vi "TCP Named Service - Server.vi"() -> ()   [LabVIEW 2013]
doc: "创建一个命名服务并在第一个可用端口侦听。当客户端连接该服务时，将发送一个响应字符串至客户端。"
panel:
  in  "发送的消息":string="当前正从客户端%s（端口%d）访问TCP Named Service - Server.vi。"
  in  "停止":bool
  # "概述：演示使用TCP函数初始化可向客户端VI发送数据的命名TCP服务。\n操作步骤：\n1. 运行VI。\n2. 打开TCP Named Service - Client.vi并按前面板上的说明操作。\n3. 单击停止可停止VI。"
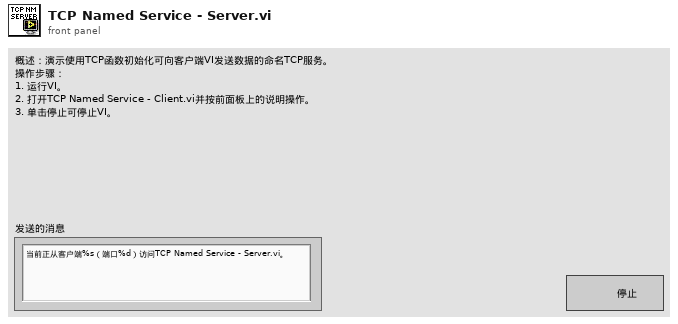
[diagram p1: front panel]
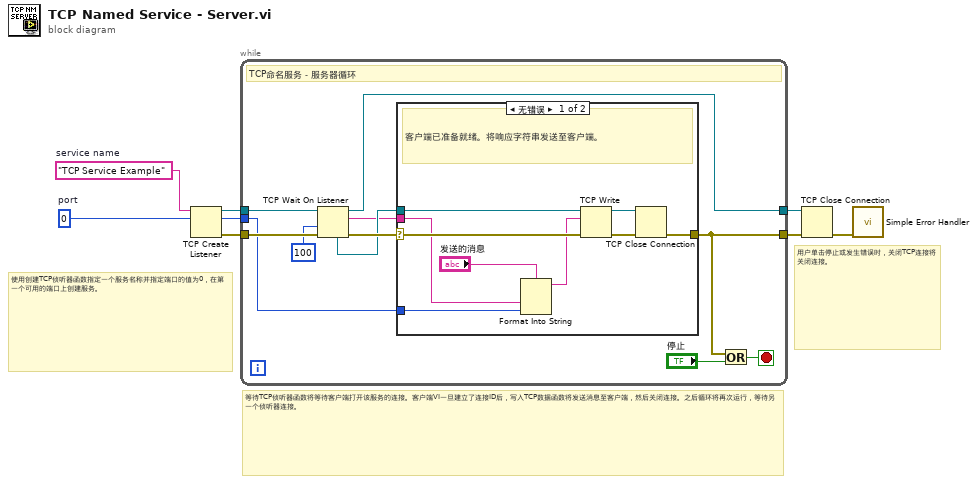
[diagram p0: block diagram]
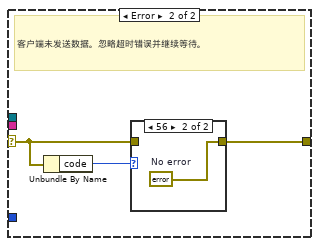
[diagram p2: hidden frame]
diagram:
  w2 = u16 0  # port
  w1 = "TCP Service Example"  # service name
  # "用户单击停止或发生错误时，关闭TCP连接将关闭连接。"
  # "等待TCP侦听器函数将等待客户端打开该服务的连接。客户端VI一旦建立了连接ID后，写入TCP数据函数将发送消息至客户端，然后关闭连接。之后循环将再次运行，等待另一个侦听器连接。"
  # "使用创建TCP侦听器函数指定一个服务名称并指定端口的值为0，在第一个可用的端口上创建服务。"
  n1 = TCP Create Listener(10:w2, 11:w1) -> (0:w7:errorcluster, 2:w4:u16, 3:w8:refnum<k5>)  [unwired: 3 in]
  n2 = while {
    tunnel: [w12] -> w5
    tunnel: w8 -> [w19]
    tunnel: w7 -> [w17]
    tunnel: [w9] -> w6
    tunnel: w4 -> [w15]
    stop <- w14 stop-if-true
    # "TCP命名服务－服务器循环"
    n3 = TCP Wait On Listener(8:w17, 9:100 ("timeout ms (25000)"), 11:w19) -> (0:w18:errorcluster, 2:w10:string, 3:w9:refnum<k5>, 4:w16:refnum<k5>)  [unwired: 1 in, 1 out]
    n4 = case shown="无错误" w18 {
      selector: w18 -> [w28 w31]
      tunnel: [w21 w29] -> w12
      tunnel: w16 -> [w22 _]
      tunnel: w15 -> [w26 _]
      tunnel: w10 -> [w24 _]
      frame No Error {
        # "客户端已准备就绪。将响应字符串发送至客户端。"
        n5 = Format Into String(format string="发送的消息", w24, w26) -> (resulting string=w23:string)  [unwired: 2 in, 1 out]
        n6 = TCP Write(connection ID=w22, data in=w23, error in (no error)=w28) -> (connection ID out=w20:refnum<k5>, error out=w27:errorcluster)  [unwired: 1 in, 1 out]
        n7 = TCP Close Connection(connection ID=w20, error in (no error)=w27) -> (error out=w21:errorcluster)  [unwired: 1 in, 1 out]
      }
      frame Error {
        # "客户端未发送数据。忽略超时错误并继续等待。"
        n8 = Unbundle By Name(w31) -> ("code"=w30:i32)
        n9 = case shown="56" w30 {
          tunnel: w31 -> [w32 _]
          tunnel: [w32 w33] -> w29
          frame Default {
          }
          frame 56 {
            w33 = errorcluster {"status"=FALSE, "code"=0, "source"=""}  # No error
          }
        }
      }
    }
    n10 = Or(x=w12, y="停止") -> (x .or. y?=w14:bool)
  }
  n11 = TCP Close Connection(connection ID=w6, error in (no error)=w5) -> (error out=w3:errorcluster)  [unwired: 1 in, 1 out]
  n12 = call <vilib>:"Simple Error Handler.vi"("error in (no error)"=w3) -> ()  [unwired: 4 in, 5 out]
